vi "Acq2.vi"() -> (3 "cos(x)":dbl)   [LabVIEW 2020]
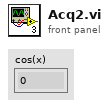
[diagram p1: front panel]
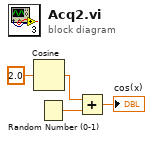
[diagram p0: block diagram]
diagram:
  n1 = Cosine(x=2.0) -> (cos(x)=w2:dbl)
  n2 = Random Number (0-1)() -> (number: 0 to 1=w3:dbl)
  n3 = Add(x=w2, y=w3) -> (x+y=→"cos(x)":dbl)
